vi "f_file vi test.vi"() -> ()   [LabVIEW 2016]
panel:
  in  "folder and file name Cluster":T1={"Path"=path "D:/Gantry_General/Main/ms_kao", "folder name"="data", "file name"="data_", "extension"="txt", "add time string"=FALSE}
  in  "2D data":dbl[][](array[numeric])=[[0.0, 1.0, 0.0], [0.0, 0.0, 2.0], [0.0, 4.0, 1.0]]
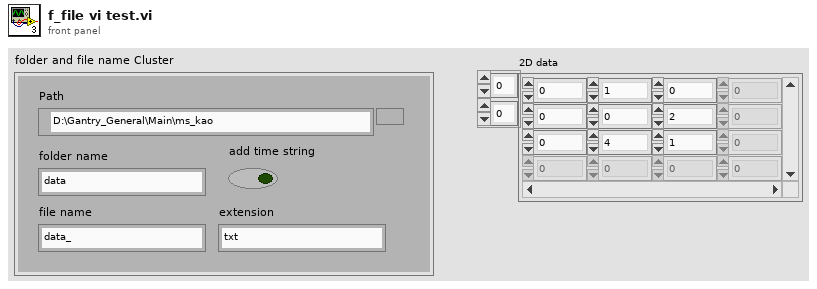
[diagram p1: front panel]
types:
  T1 = cluster{"Path":path, "folder name":string, "file name":string, "extension":string, "add time string":bool}
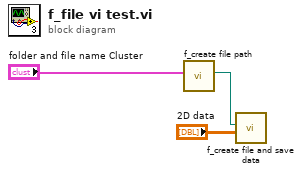
[diagram p0: block diagram]
diagram:
  n1 = call "f_create file path.vi"("folder and file name Cluster"="folder and file name Cluster") -> ("appended path"=w3:path)  [unwired: 10 in]
  n2 = call "f_create file and save data.vi"("2D data"="2D data", "path"=w3) -> ()  [unwired: 10 in]
